vi "DestroyPublicEvents.vi"(8 "error in (no error)":errorcluster, 11 "Inst.MOTOR":refnum<class "Inst.MOTOR.lvclass">) -> (0 "error out":errorcluster, 3 "Inst.MOTOR out":refnum<class "Inst.MOTOR.lvclass">)   [LabVIEW 2019, in "Inst.MOTOR.lvclass"]
doc: "JKI State Machine Objects (SMO) 1.0.0.5\nJKI - JKI\nCopyright (c) 2016, JKI"
uses:
  Inst.MOTOR.lvclass
  <userlib>/LevyLab/Instrument Framework/Instrument Types/VSource/Instrument.VSource.lvclass
panel:
  # "For instructions on how to use the JKI State Machine Objects, examples and video tutorials, visit:\nhttp://jki.net/state-machine-objects/\n\nJKI State Machine Objects™\nhttp://jki.net/state-machine-objects/\nCopyright (C) 2005-2015, JKI <info@jki.net>\nALL RIGHTS RESERVED"
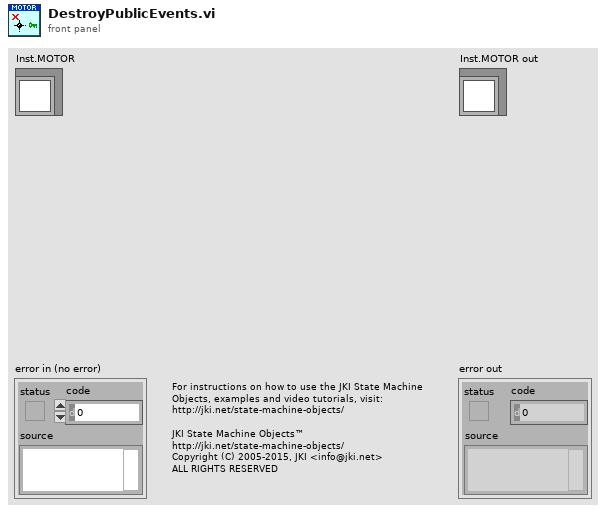
[diagram p1: front panel]
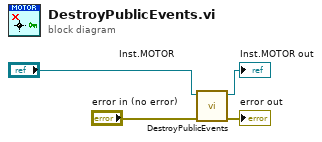
[diagram p0: block diagram]
diagram:
  n1 = call-parent "DestroyPublicEvents.vi"("error in (no error)"="error in (no error)", "Instrument"="Inst.MOTOR") -> ("error out"=→"error out":errorcluster, "Instrument out"=→"Inst.MOTOR out":refnum<class "Inst.MOTOR.lvclass">)  [unwired: 8 in]
